vi "Abort Iterations.vi"(8 "error in (no error)":errorcluster, 11 "Function in":refnum<class "Function.lvclass">) -> (0 "error out":errorcluster, 3 "Function out":refnum<class "Function.lvclass">)   [LabVIEW 2016]
uses:
  <userlib>/Common Components/Function Actor/Function.lvclass
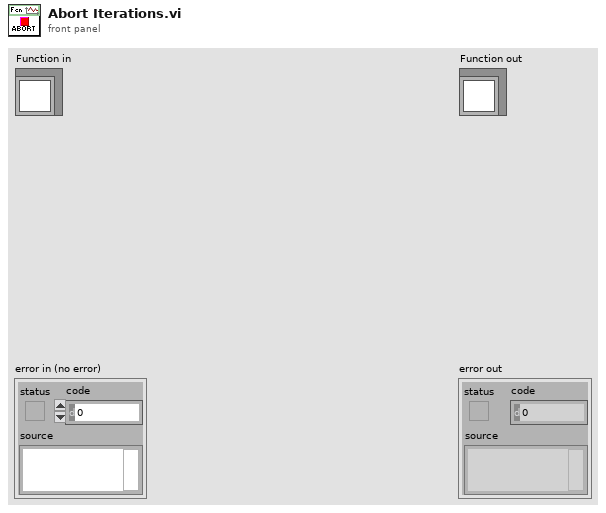
[diagram p1: front panel]
types:
  T1 = typedef "Iteration Count.ctl" = cluster{"Desired Iterations":i32, "Current":i32}
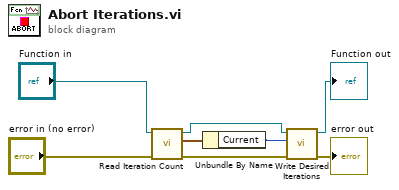
[diagram p0: block diagram]
diagram:
  n1 = call <userlib>:"Read Iteration Count.vi"("error in (no error)"="error in (no error)", "Function in"="Function in") -> ("error out"=w7:errorcluster, "Iteration Count"=w2:T1, "Function out"=w4:refnum<class "Function.lvclass">)  [unwired: 7 in]
  n2 = Unbundle By Name(w2) -> ("Current"=w1:i32)
  n3 = call <userlib>:"Write Desired Iterations.vi"("error in (no error)"=w7, "Desired Iterations"=w1, "Function in"=w4) -> ("error out"=→"error out":errorcluster, "Function out"=→"Function out":refnum<class "Function.lvclass">)  [unwired: 7 in]
